vi "Request Data JSON.vi"(8 "error in (no error)":errorcluster, 11 "SetCurrentSceneCollection in":refnum<class "SetCurrentSceneCollection.lvclass">) -> (0 "error out":errorcluster, 2 "Request Data JSON":string, 3 "SetCurrentSceneCollection out":refnum<class "SetCurrentSceneCollection.lvclass">)   [LabVIEW 2020, in "obs-websocket.lvlib" / "SetCurrentSceneCollection.lvclass"]
uses:
  SetCurrentSceneCollection.lvclass
  SetCurrentSceneCollection.lvclass/SetCurrentSceneCollection.ctl
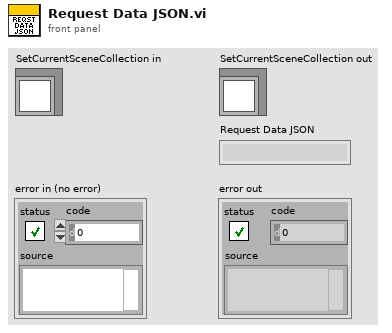
[diagram p1: front panel]
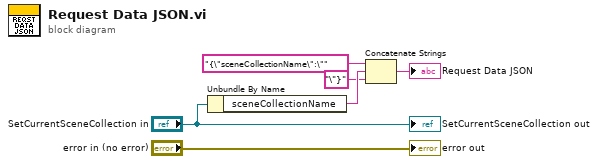
[diagram p0: block diagram]
diagram:
  n1 = Unbundle By Name("SetCurrentSceneCollection in") -> ("sceneCollectionName"=w3:string)
  n2 = Concatenate Strings("{\"sceneCollectionName\":\"" ("string"), w3, "\"}" ("string")) -> (→"Request Data JSON":string)
  "error out" <- "error in (no error)"
  "SetCurrentSceneCollection out" <- "SetCurrentSceneCollection in"
